vi "CAN-LIN Frame Generator_client.vi"() -> ()   [LabVIEW 2025]
uses:
  can-lin/CAN-LIN Raw Bus Capture UI/OOB gRPC Client/RPC Messages/hwval_BoolRequest.ctl
  can-lin/CAN-LIN Raw Bus Capture UI/OOB gRPC Client/RPC Messages/hwval_ExportRequest.ctl
  can-lin/CAN-LIN Raw Bus Capture UI/OOB gRPC Client/RPC Messages/hwval_GenericRequest.ctl
  can-lin/CAN-LIN Raw Bus Capture UI/OOB gRPC Client/OOB gRPC Client.lvlib
panel:
  in  "stop":bool
  in  "Export":bool
  in  "Export File Type":string(combo)="RAW"
  in  "STOP":bool
  in  "PauseResume":bool caption="Pause"
  in  "OOB gRPC Port":i32
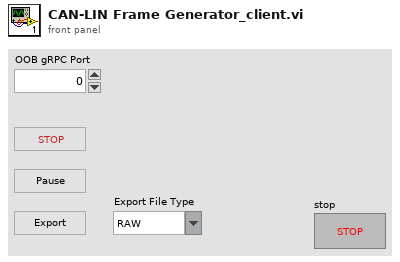
[diagram p1: front panel]
types:
  T1 = typedef "grpc-lvsupport-release.lvlib/grpcId.ctl" = u64
  T2 = typedef "OOB gRPC Client.lvlib/hwval_BoolRequest.ctl" = cluster{"BooleanData":bool}
  T3 = typedef "OOB gRPC Client.lvlib/hwval_ExportRequest.ctl" = cluster{"FileType":string}
  T4 = typedef "OOB gRPC Client.lvlib/hwval_GenericRequest.ctl" = cluster{"Command":string, "Payload":u8[]}
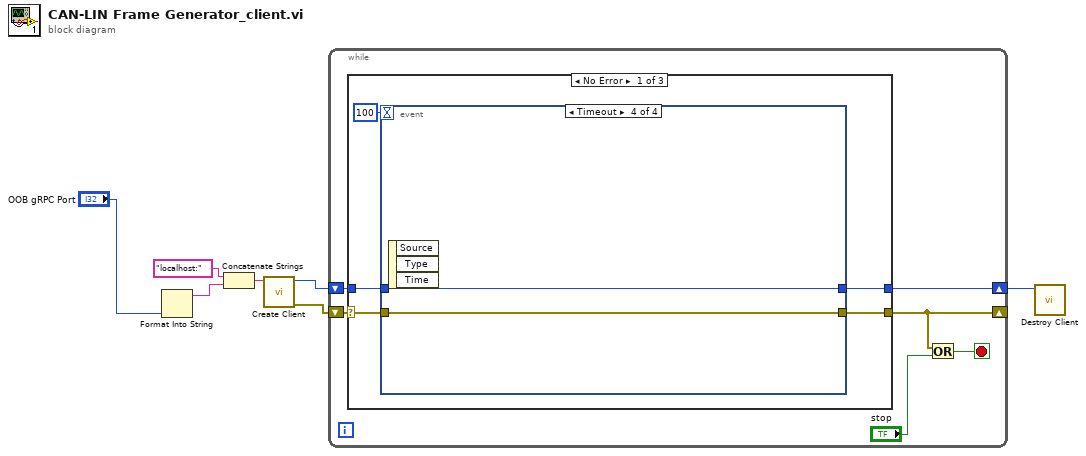
[diagram p0: block diagram]
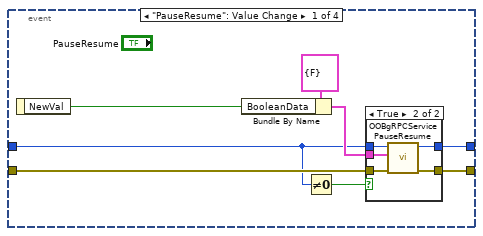
[diagram p2: hidden frame]
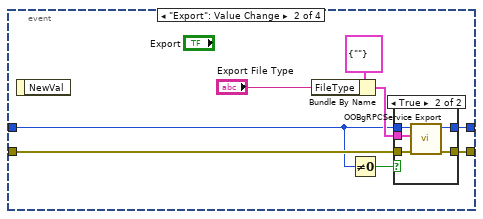
[diagram p4: hidden frame]
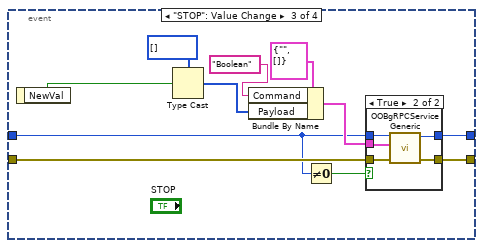
[diagram p6: hidden frame]
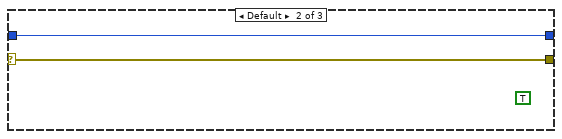
[diagram p8: hidden frame]
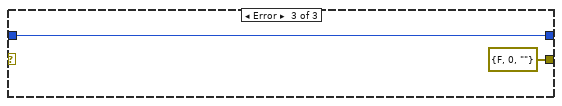
[diagram p9: hidden frame]
diagram:
  n1 = Format Into String("OOB gRPC Port") -> (resulting string=w7:string)  [unwired: 3 in, 1 out]
  n2 = Concatenate Strings("localhost:" ("string"), w7) -> (w5:string)
  n3 = call "Create Client.vi"("address"=w5) -> ("error out"=w2:errorcluster, "gRPC ID Out"=w3:T1)  [unwired: 9 in]
  n4 = while {
    shift-right: [w8] -> _
    shift-left: w2 -> [w13]
    shift-right: [w11] -> w1
    shift-left: w3 -> [w12]
    stop <- w10 stop-if-true
    n5 = case shown="No Error" w13 {
      selector: w13 -> [w17 w69 _]
      tunnel: [w18 w69 errorcluster {"status"=FALSE, "code"=0, "source"=""} ("error IO")] -> w8
      tunnel: w12 -> [w16 w70 w71]
      tunnel: [w15 w70 w71] -> w11
      frame No Error {
        n6 = event shown="[3] Timeout" {
          selector: _ -> [_ _ _ _]
          dyn-events: _ -> [_ _ _ _]
          timeout: 100 -> [_ _ _ _]
          tunnel: [w25 w40 w58 w67] -> w18
          tunnel: w17 -> [w24 w39 w57 w67]
          tunnel: w16 -> [w19 w35 w54 w68]
          tunnel: [w26 w41 w59 w68] -> w15
          event "PauseResume": Value Change {
            n7 = event-data() -> ("NewVal"=w21:bool)  [unwired: 1 in]
            n8 = Bundle By Name(cluster=T2 {"BooleanData"=FALSE} ("Request Data"), "BooleanData"=w21) -> (w22:T2)
            n9 = Not Equal To 0?(x=w19) -> (x != 0?=w20:bool)
            n10 = case shown="True" w20 {
              tunnel: [w28 w33] -> w26
              tunnel: [w27 w32] -> w25
              tunnel: w19 -> [w28 w31]
              tunnel: w24 -> [w27 w30]
              tunnel: w22 -> [_ w29]
              frame False {
              }
              frame True {
                n11 = call "OOBgRPCService PauseResume.vi"("error in"=w30, "Request Data"=w29, "gRPC ID"=w31) -> ("error out"=w32:errorcluster, "gRPC ID out"=w33:T1)  [unwired: 6 in, 1 out]
              }
            }
          }
          event "Export": Value Change {
            n12 = event-data() -> ()  [unwired: 1 in, 1 out]
            n13 = Bundle By Name(cluster=T3 {"FileType"=""} ("Request Data"), "FileType"="Export File Type") -> (w37:T3)
            n14 = Not Equal To 0?(x=w35) -> (x != 0?=w36:bool)
            n15 = case shown="True" w36 {
              tunnel: [w43 w48] -> w41
              tunnel: [w42 w47] -> w40
              tunnel: w35 -> [w43 w46]
              tunnel: w39 -> [w42 w45]
              tunnel: w37 -> [_ w44]
              frame False {
              }
              frame True {
                n16 = call "OOBgRPCService Export.vi"("error in"=w45, "Request Data"=w44, "gRPC ID"=w46) -> ("error out"=w47:errorcluster, "gRPC ID out"=w48:T1)  [unwired: 6 in, 1 out]
              }
            }
          }
          event "STOP": Value Change {
            n17 = event-data() -> ("NewVal"=w51:bool)  [unwired: 1 in]
            n18 = Type Cast(type=u8[] [] ("Payload"), x=w51) -> (*(type *) &x=w50:u8[])
            n19 = Bundle By Name(cluster=T4 {"Command"="", "Payload"=[]} ("Request Data"), "Command"="Boolean", "Payload"=w50) -> (w56:T4)
            n20 = Not Equal To 0?(x=w54) -> (x != 0?=w55:bool)
            n21 = case shown="True" w55 {
              tunnel: [w61 w65] -> w59
              tunnel: [w60 w64] -> w58
              tunnel: w54 -> [w61 w66]
              tunnel: w57 -> [w60 w63]
              tunnel: w56 -> [_ w62]
              frame False {
              }
              frame True {
                n22 = call "OOBgRPCService Generic.vi"("error in"=w63, "Request Data"=w62, "gRPC ID"=w66) -> ("error out"=w64:errorcluster, "gRPC ID out"=w65:T1)  [unwired: 6 in, 1 out]
              }
            }
          }
          event Timeout {
            n23 = event-data() -> ()  [unwired: 1 in, 3 out]
          }
        }
      }
      frame Default {
        (unwired) TRUE
      }
      frame Error {
      }
    }
    n24 = Or(x=w8, y="stop") -> (x .or. y?=w10:bool)
  }
  n25 = call "Destroy Client.vi"("gRPC ID"=w1) -> ()  [unwired: 10 in, 1 out]
